vi "Find Resource by Type (String).vi"(6 "Error if not found? (F)":bool, 8 "error in (no error)":errorcluster, 10 "Resource Type":string, 11 "Resources":T1[](array[typedef])) -> (0 "error out":errorcluster, 1 "Index":i32, 2 "Resource":T1, 3 "Resources out":T1[](array[typedef]), 5 "Found?":bool)   [LabVIEW 2026, in "VILab.lvlib"]
uses:
  VILab.lvlib
  CTLs/Resource.ctl
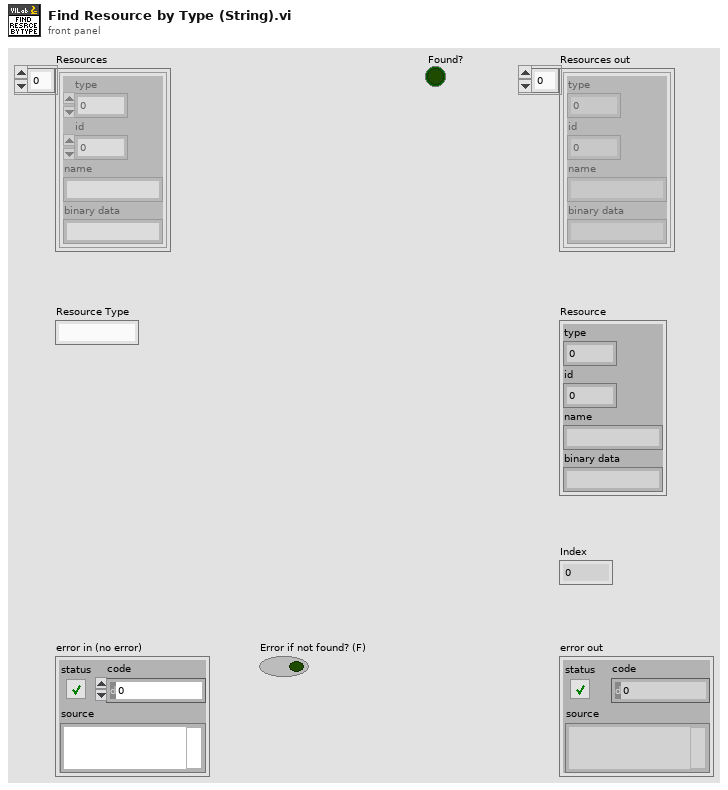
[diagram p1: front panel]
types:
  T1 = typedef "VILab.lvlib/Resource.ctl" = cluster{"type":u32, "id":i32, "name":string, "binary data":string}
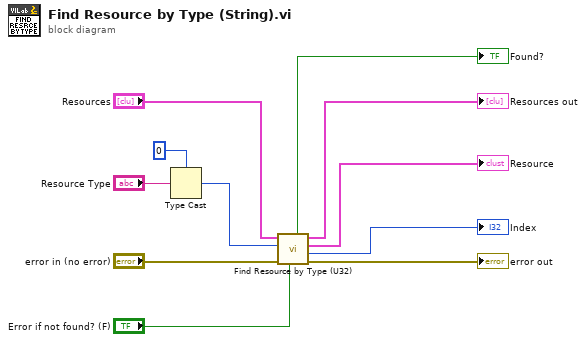
[diagram p0: block diagram]
diagram:
  n1 = Type Cast(type=u32 0 ("Resource Type"), x="Resource Type") -> (*(type *) &x=w8:u32)
  n2 = call "Find Resource by Type (U32).vi"("Error if not found? (F)"="Error if not found? (F)", "error in (no error)"="error in (no error)", "Resource Type"=w8, "Resources"="Resources") -> ("error out"=→"error out":errorcluster, "Index"=→"Index":i32, "Resource"=→"Resource":T1, "Resources out"=→"Resources out":T1[], "Found?"=→"Found?":bool)  [unwired: 3 in]
